vi "d calc w y.vi"(7 "y p":dbl) -> (5 "d":dbl)   [LabVIEW 2016]
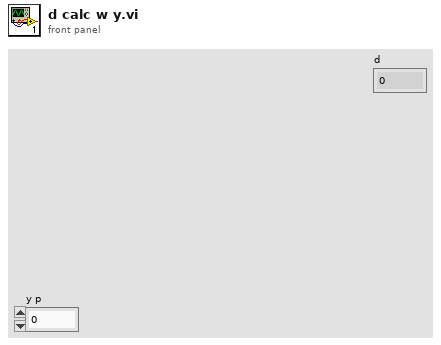
[diagram p1: front panel]
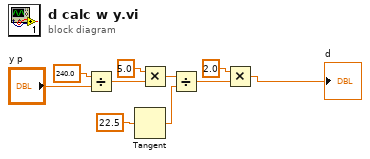
[diagram p0: block diagram]
diagram:
  n1 = Divide(x=240.0 ("y"), y="y p") -> (x/y=w5:dbl)
  n2 = Tangent(1:22.5 ("x")) -> (0:w7:dbl)
  n3 = Multiply(x=5.0, y=w5) -> (x*y=w4:dbl)
  n4 = Divide(x=w4, y=w7) -> (x/y=w8:dbl)
  n5 = Multiply(x=2.0, y=w8) -> (x*y=→"d":dbl)
